vi "Subscribe.vi"(8 "error in (no error)":errorcluster, 9 "Event Name":string, 10 "Cell#":string, 11 "connection in":T1) -> (0 "error out":errorcluster, 3 "connection out":T1)   [LabVIEW 2013, in "FRCts20_SNS.lvlib"]
uses:
  FRCts20_SNS.lvlib
  Perforce/penguin_1666/mblack_PerforceWin/lvdotcom/source/aws-toolkit/r1/trunk/SNS/VI Source/AWS SNS Class/AWS_SNS.lvclass
  <vilib>/National Instruments/LabVIEW Interface for Amazon S3/Typedefs/AMZ_S3_AWS Credentials.ctl
  <vilib>/National Instruments/LabVIEW Interface for Amazon S3/LV Interface for Amazon S3.lvlib
  Perforce/penguin_1666/mblack_PerforceWin/lvdotcom/source/aws-toolkit/r1/trunk/SNS/VI Source/Public Typedefs/AWS_SNS Subcribe Parameters.ctl
  Perforce/penguin_1666/mblack_PerforceWin/lvdotcom/source/aws-toolkit/r1/trunk/SNS/VI Source/AWS_SNS.lvlib
  <vilib>/addons/database/NI_Database_API.lvlib
  <vilib>/addons/database/Connection.llb/DB Tools Open Connec (String).vi
  <vilib>/addons/database/Connection.llb/Conn ObjectReference.ctl
panel:
  # "1-XXX-XXX-XXXX"
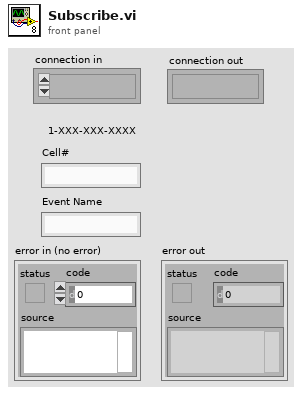
[diagram p1: front panel]
types:
  T1 = typedef "NI_Database_API.lvlib/Conn ObjectReference.ctl" = refnum<k1>
  T2 = typedef "AWS_SNS.lvlib/AWS_SNS Subcribe Parameters.ctl" = cluster{"Endpoint":string, "Protocol":string, "TopicArn":string}
  T3 = typedef "LV Interface for Amazon S3.lvlib/AMZ_S3_AWS Credentials.ctl" = cluster{"Access Key":string, "Secret Key":string}
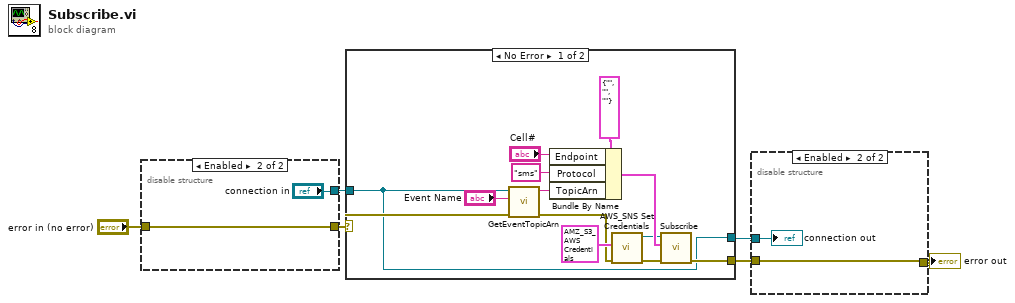
[diagram p0: block diagram]
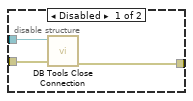
[diagram p2: hidden frame]
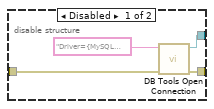
[diagram p3: hidden frame]
diagram:
  n1 = disable-structure shown="Enabled" {
    disable-tunnel: "error in (no error)" -> [w9 w11]
    disable-tunnel: [w8 w11] -> w5
    disable-tunnel: [w7 "connection in"] -> w4
    frame Disabled {
      n2 = call-poly <vilib>:"DB Tools Open Connection.vi"("error in (no error)"=w9, "connection information"="Driver={MySQL ODBC 5.2w Driver};Server=parkway-test-db.cjlclmebggwl.us-east-1.rds.amazonaws.com;Database=parkway;User=parkway;Password=moonlightmarj" ("Connection String")) -> ("error out"=w8:errorcluster, "connection reference"=w7:T1)  [unwired: 6 in]
    }
    frame Enabled {
    }
  }
  n3 = case shown="No Error" w5 {
    selector: w5 -> [w15 w27]
    tunnel: [w16 w27] -> w2
    tunnel: w4 -> [w13 w26]
    tunnel: [w13 w26] -> w3
    frame No Error {
      n4 = call "GetEventTopicArn.vi"("error in (no error)"=w15, "Event Name"="Event Name", "Refnum in"=w13) -> ("error out"=w14:errorcluster, "TopicArn"=w17:string)  [unwired: 7 in]
      n5 = Bundle By Name(cluster=T2 {"Endpoint"="", "Protocol"="", "TopicArn"=""} ("Subscribe Parameters"), "Endpoint"="Cell#", "Protocol"="sms", "TopicArn"=w17) -> (w25:T2)
      n6 = call "AWS_SNS Set Credentials.vi"("error in (no error)"=w14, "AWS Credentials"=T3 {"Access Key"="AKIAI4UOFGXQQ2XM3KTQ", "Secret Key"="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"} ("AWS Credentials in")) -> ("error out"=w21:errorcluster, "AWS_SNS.lvlib:AWS_SNS.lvclass"=w20:refnum<class "AWS_SNS.lvclass">)  [unwired: 8 in]
      n7 = call-dynamic "Subscribe.vi"("error in (no error)"=w21, "Subscribe Parameters"=w25, "AWS_SNS.lvlib:AWS_SNS.lvclass"=w20) -> ("error out"=w16:errorcluster)  [unwired: 6 in, 2 out]
    }
    frame Error {
    }
  }
  n8 = disable-structure shown="Enabled" {
    disable-tunnel: w3 -> [w30 w31]
    disable-tunnel: w2 -> [w29 w32]
    disable-tunnel: [w28 w32] -> w1
    frame Disabled {
      n9 = call <vilib>:"DB Tools Close Connection.vi"("error in (no error)"=w29, "connection reference"=w30) -> ("error out"=w28:errorcluster)  [unwired: 5 in]
    }
    frame Enabled {
      "connection out" <- w31
    }
  }
  "error out" <- w1
